vi "Highlight Item Message.vi"(6 "Item name":string, 7 "Project Name":string, 8 "error in (no error)":errorcluster, 9 "Section":string, 10 "Library Name":string, 11 "Delacor_lib_QMH_Message Queue in":refnum<class "Delacor_lib_QMH_Message Queue.lvclass">) -> (0 "error out":errorcluster)   [LabVIEW 2019, in "Panther Dashboard.lvlib"]
uses:
  Panther Dashboard.lvlib
  <vilib>/Delacor/Delacor QMH/Libraries/Message Queue_class/Delacor_lib_QMH_Message Queue.lvclass
  <vilib>/Delacor/Delacor QMH/Libraries/Message Queue_class/Delacor_lib_QMH_Enqueue Message (Single).vi
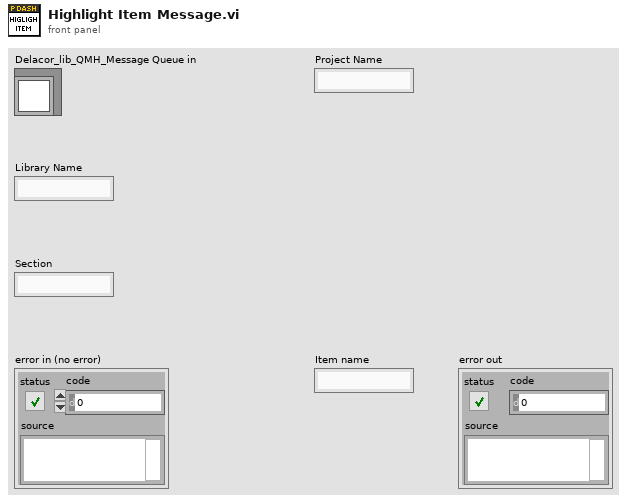
[diagram p1: front panel]
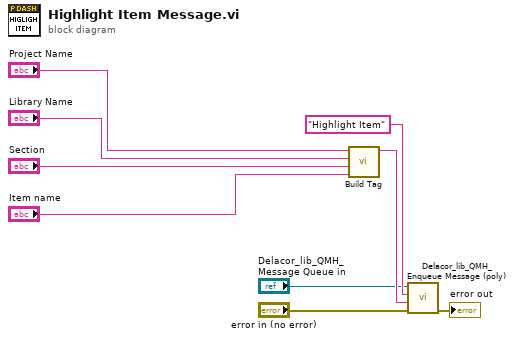
[diagram p0: block diagram]
diagram:
  n1 = call "Build Tag.vi"("Item"="Item name", "Section"="Section", "Library Name"="Library Name", "Project Name"="Project Name") -> ("Tag"=w9:string)  [unwired: 7 in]
  n2 = call-poly <vilib>:"Delacor_lib_QMH_Enqueue Message (poly).vi"("error in"="error in (no error)", "Message Data"=w9, "Message"="Highlight Item", "Message Queue in"="Delacor_lib_QMH_Message Queue in") -> ("error out"=→"error out":errorcluster)  [unwired: 6 in, 1 out]
